vi "Drive Straight PID.vi"(5 "Angle Offset":dbl, 6 "Iteration":i32, 7 "target distance":dbl, 8 "Period (ms)":i64=10) -> (1 "Complete?":bool, 2 "Right Axis":dbl, 3 "Left Axis":dbl)   [LabVIEW 2018]
uses:
  Odometry/Typedef/Odometry.ctl
  <vilib>/addons/control/pid/pid.llb/PID Output Rate Limiter (DBL).vi
  <vilib>/addons/control/pid/NI_PID_pid.lvlib
panel:
  in  "Odometry":T1
  in  "output rate":dbl=80.0 format="%.2f"
  in  "Gyro PIDF":cluster{"Kp":dbl, "Ki":dbl, "Kd":dbl, "Kf":dbl}={"Kp"=0.05, "Ki"=0.0, "Kd"=0.0, "Kf"=0.0} {"Kf" format="%.3f"; "Kd" format="%.3f"; "Ki" format="%.3f"; "Kp" format="%.3f"}
  in  "PIDF":cluster{"Kp":dbl, "Ki":dbl, "Kd":dbl, "Kf":dbl}={"Kp"=0.02, "Ki"=0.0, "Kd"=0.045, "Kf"=0.0} {"Kf" format="%.3f"; "Kd" format="%.3f"; "Ki" format="%.3f"; "Kp" format="%.3f"}
  in  "i Zone":dbl=12.0 format="%.2f"
  in  "output range":cluster{"output high":dbl, "output low":dbl}={"output high"=1.0, "output low"=-1.0} {"output low" format="%.2f"; "output high" format="%.2f"}
  out "Waveform Chart 2":cluster{dbl, dbl}(graph)={-50.0, -50.00778875}
  out "Gyro Output":dbl(graph)=0.02713616249999992
  out "mean":dbl=0.00016497888749945157 format="%0.2f"
  in  "threshold":dbl=0.008
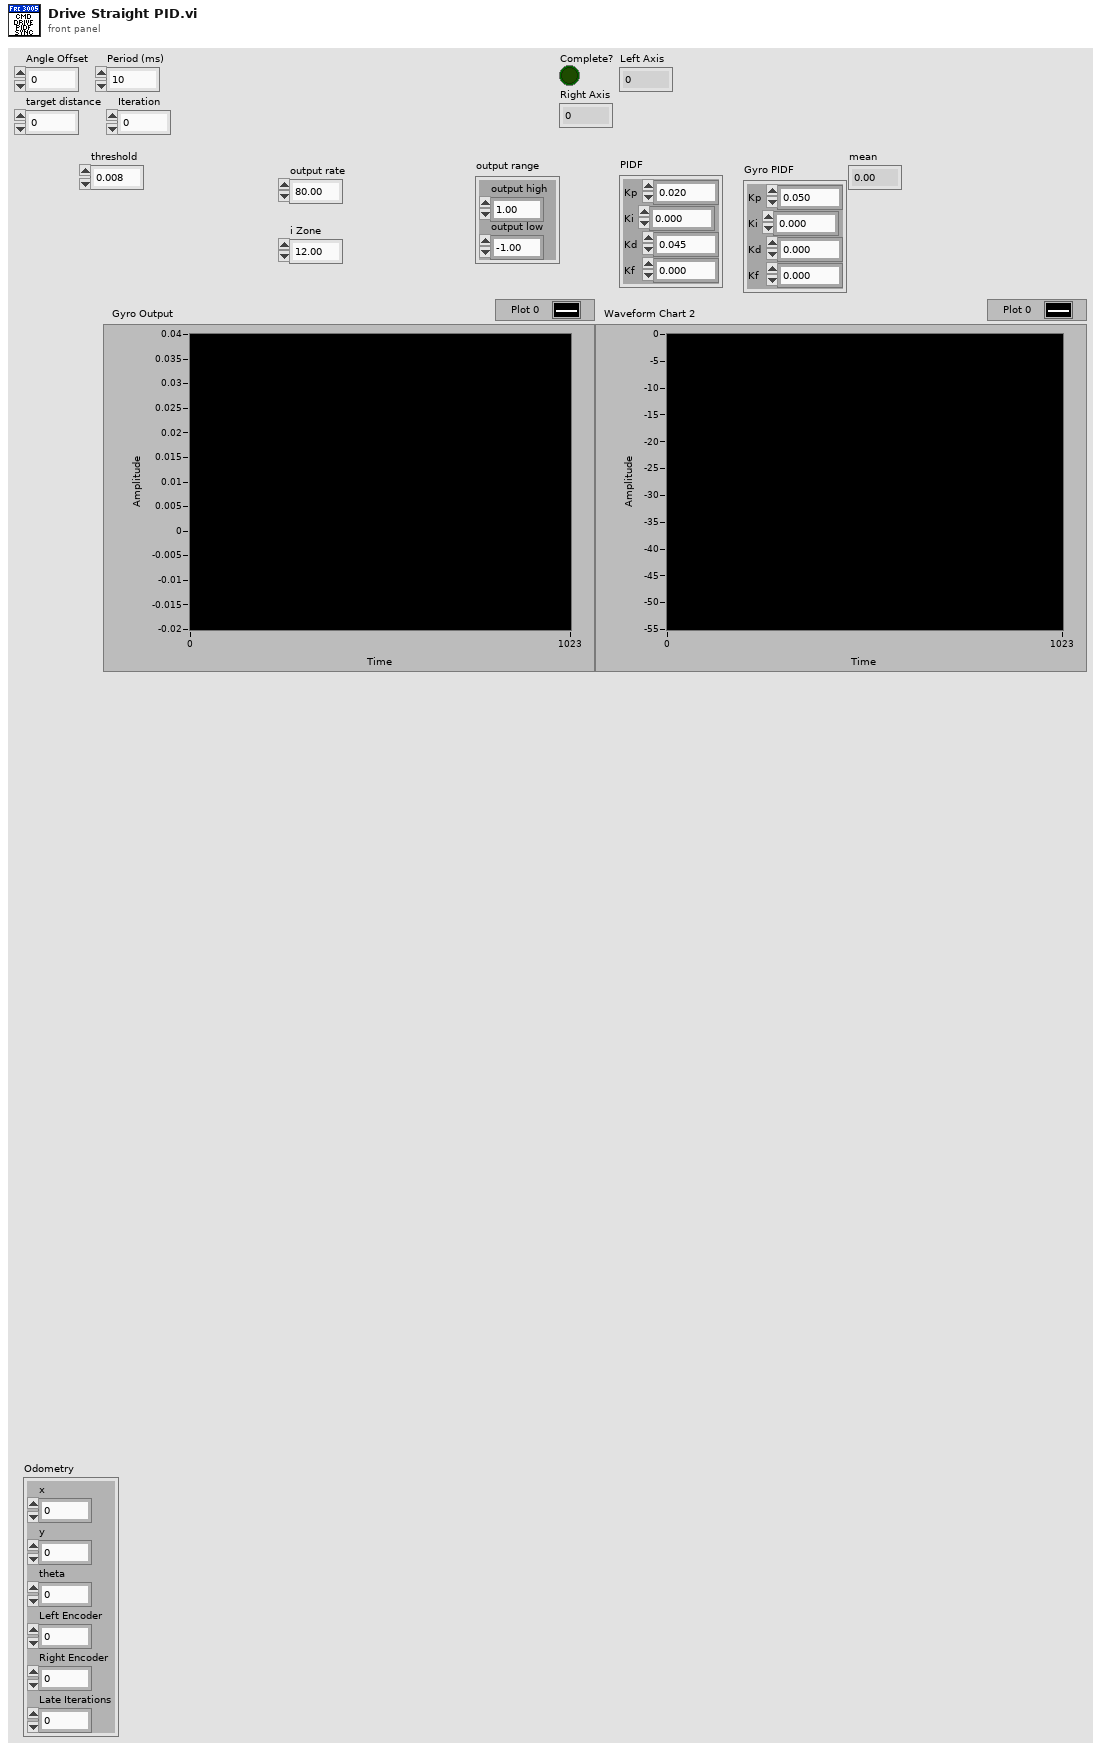
[diagram p1: front panel]
types:
  T1 = typedef "Odometry.ctl" = cluster{"x":dbl, "y":dbl, "theta":dbl, "Left Encoder":dbl, "Right Encoder":dbl, "Late Iterations":i16}
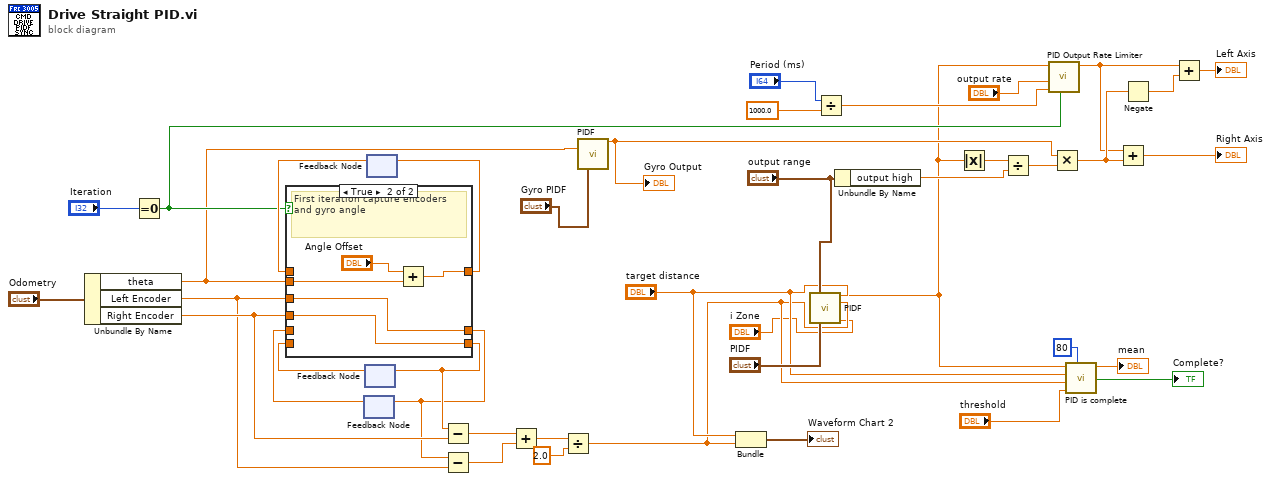
[diagram p0: block diagram]
diagram:
  n1 = Unbundle By Name("Odometry") -> ("theta"=w8:dbl, "Left Encoder"=w12:dbl, "Right Encoder"=w14:dbl)
  n2 = Equal To 0?(x="Iteration") -> (x = 0?=w24:bool)
  n3 = feedback #1() -> (w16:dbl)  [unwired: 1 in]
  n4 = feedback #2() -> (w17:dbl)  [unwired: 1 in]
  n5 = feedback #3() -> (w26:dbl)  [unwired: 1 in]
  n6 = case shown="True" w24 {
    tunnel: [w44 w48] -> w27
    tunnel: w26 -> [w44 _]
    tunnel: w8 -> [_ w47]
    tunnel: w12 -> [_ w45]
    tunnel: w14 -> [_ w46]
    tunnel: [w43 w46] -> w15
    tunnel: [w42 w45] -> w13
    tunnel: w17 -> [w43 _]
    tunnel: w16 -> [w42 _]
    frame False {
    }
    frame True {
      # "First iteration capture encoders and gyro angle"
      n7 = Add(x="Angle Offset", y=w47) -> (x+y=w48:dbl)
    }
  }
  n8 = feedback-in #1(w13) -> ()
  n9 = feedback-in #2(w15) -> ()
  n10 = feedback-in #3(w27) -> ()
  n11 = Subtract(x=w15, y=w14) -> (x-y=w11:dbl)
  n12 = Subtract(x=w13, y=w12) -> (x-y=w10:dbl)
  n13 = Add(x=w11, y=w10) -> (x+y=w41:dbl)
  n14 = Divide(x=w41, y=2.0) -> (x/y=w3:dbl)
  n15 = call "PIDF.vi"("process variable"=w8, "PIDF gains"="Gyro PIDF") -> ("output"=w7:dbl)  [unwired: 11 in, 2 out]
  "Gyro Output" <- w7
  n16 = Bundle("target distance"="target distance", w3) -> (→"Waveform Chart 2":cluster{"target distance":dbl, dbl})  [unwired: 1 in]
  n17 = call "PIDF.vi"("setpoint"="target distance", "output range"="output range", "process variable"=w3, "i Zone"="i Zone", "PIDF gains"="PIDF") -> ("output"=w1:dbl)  [unwired: 8 in, 2 out]
  n18 = Divide(x="Period (ms)", y=1000.0) -> (x/y=w37:dbl)
  n19 = Unbundle By Name("output range") -> ("output high"=w33:dbl)
  n20 = Absolute Value(x=w1) -> (abs(x)=w20:dbl)
  n21 = Divide(x=w20, y=w33) -> (x/y=w32:dbl)
  n22 = call-poly <vilib>:"PID Output Rate Limiter.vi"("reinitialize? (F)"=w24, "dt (s)"=w37, "output rate (EGU/min)"="output rate", "input (controller output)"=w1) -> ("output"=w29:dbl)  [unwired: 4 in, 1 out]
  n23 = Multiply(x=w7, y=w32) -> (x*y=w34:dbl)
  n24 = call "PID is complete.vi"("sample length"=80, "threshold"="threshold", "process variable"=w3, "setpoint"="target distance", "PID Output"=w1) -> ("PID is Done?"=→"Complete?":bool, "mean"=→"mean":dbl)  [unwired: 5 in]
  n25 = Add(x=w29, y=w34) -> (x+y=→"Right Axis":dbl)
  n26 = Negate(x=w34) -> (-x=w35:dbl)
  n27 = Add(x=w29, y=w35) -> (x+y=→"Left Axis":dbl)
